vi "test Check If Custom Device is Enabled.vi"(8 "error in":errorcluster, 11 "TestCase in":refnum<class "Scripting.lvclass">) -> (0 "error out":errorcluster)   [LabVIEW 2020, in "Scripting.lvclass"]
uses:
  Scripting.lvclass
  <vilib>/addons/_JKI Toolkits/VI Tester/TestCase.llb/TestCase.lvclass
  Scripting/AIM/AIM ARINC 429 Scripting.lvlib
  C:/Program Files (x86)/National Instruments/LabVIEW 2020/vi.lib/addons/_JKI Toolkits/VI Tester/TestCase.llb/TestCase.lvclass
  C:/dev/git/niveristand-aim-arinc429-custom-device/Source/Custom Device Support/Tests/Unit/Scripting/Scripting.lvclass
panel:
  out "TestCase out":refnum<class "Scripting.lvclass">
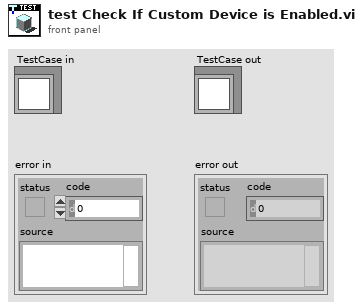
[diagram p1: front panel]
types:
  T1 = typedef "Custom Device API.lvlib/Custom Device Item Ref.ctl" = u64
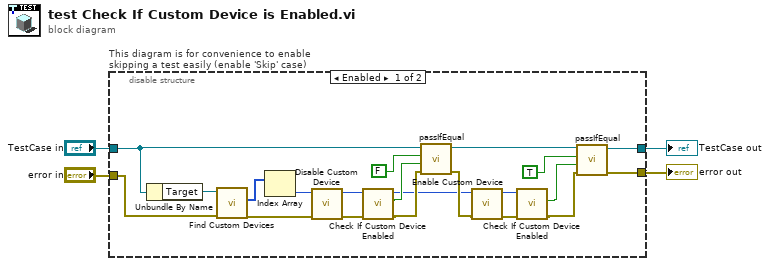
[diagram p0: block diagram]
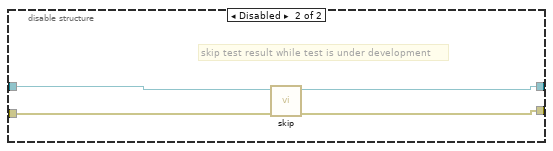
[diagram p2: hidden frame]
diagram:
  n1 = disable-structure "This diagram is for convenience to enable skipping a test easily (enable 'Skip' case)" shown="Enabled" {
    disable-tunnel: "TestCase in" -> [w25 w29]
    disable-tunnel: [w21 w27] -> w1
    disable-tunnel: [w22 w28] -> w3
    disable-tunnel: "error in" -> [w16 w26]
    frame Enabled {
      n2 = Unbundle By Name(w25) -> ("Target"=w17:refnum<k24>)
      n3 = call "Find Custom Devices.vi"("error in"=w16, "target"=w17) -> ("error out"=w13:errorcluster, "AIM ARINC 429 custom devices"=w15:u64[])  [unwired: 7 in, 1 out]
      n4 = Index Array(array=w15) -> (element=w14:u64)  [unwired: 1 in]
      n5 = call "Disable Custom Device.vi"("error in (no error)"=w13, "AIM ARINC 429 ref"=w14) -> ("error out"=w12:errorcluster, "AIM ARINC 429 ref out"=w11:T1)  [unwired: 8 in]
      n6 = call "Check If Custom Device Enabled.vi"("error in (no error)"=w12, "AIM ARINC 429 ref"=w11) -> ("error out"=w10:errorcluster, "Is Custom Device Enabled?"=w9:bool, "AIM ARINC 429 ref"=w7:T1)  [unwired: 7 in]
      n7 = call-dynamic "passIfEqual.vi"("error in (no error)"=w10, "y"=w9, "x"=FALSE, "TestCase in"=w25) -> ("error out"=w8:errorcluster, "TestCase out"=w20:refnum<class "Scripting.lvclass">)  [unwired: 6 in]
      n8 = call "Enable Custom Device.vi"("error in (no error)"=w8, "AIM ARINC 429 ref"=w7) -> ("error out"=w19:errorcluster, "AIM ARINC 429 ref out"=w18:T1)  [unwired: 8 in]
      n9 = call "Check If Custom Device Enabled.vi"("error in (no error)"=w19, "AIM ARINC 429 ref"=w18) -> ("error out"=w6:errorcluster, "Is Custom Device Enabled?"=w5:bool)  [unwired: 7 in, 1 out]
      n10 = call-dynamic "passIfEqual.vi"("error in (no error)"=w6, "y"=w5, "x"=TRUE, "TestCase in"=w20) -> ("error out"=w22:errorcluster, "TestCase out"=w21:refnum<class "Scripting.lvclass">)  [unwired: 6 in]
    }
    frame Disabled {
      # "skip test result while test is under development"
      n11 = call <vilib>:"skip.vi"("error in (no error)"=w26, "TestCase in"=w29) -> ("error out"=w28:errorcluster, "TestCase out"=w27:refnum<class "Scripting.lvclass">)  [unwired: 8 in]
    }
  }
  "error out" <- w3
  "TestCase out" <- w1
